vi "TCP Connection Manager.vi"(0 "TCP Ref":T1, 5 "Connection In":T3, 7 "Index":i32, 9 "Method":T5, 11 "error in (no error)":errorcluster, 12 "Properties In":T2) -> (3 "All Properties":T2[](array[typedef]), 4 "TCP Ref out":T1, 6 "Connection Out":T3, 8 "All Connections":T3[](array[typedef]), 10 "Number of Connections":i32, 14 "Properties out":T2, 15 "error out":errorcluster)   [LabVIEW 2013, in "J1939 Addon Shared.lvlib"]
doc: "This VI maintains the list of host connections."
uses:
  J1939 Addon Shared.lvlib
  stm_TCPConnectionMethod.ctl
  TCP/stm_TCP Connection Info.ctl
  _SubVIs/stm_MetaDataElement.ctl
  stm_TCPConnectionProperties.ctl
  J1939 Multi Packet Frame/Types/RQST Comm Lookup Table_Ref.ctl
  stm_ManagerStateVariables.ctl
  Engine/J1939 Addon Engine.lvlib
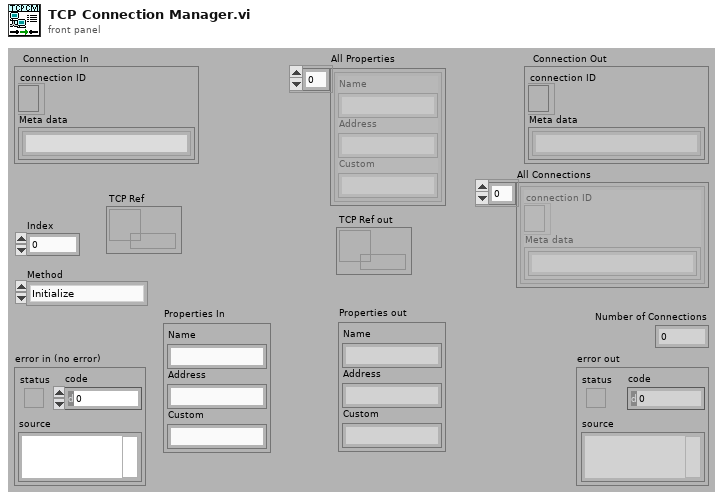
[diagram p1: front panel]
types:
  T1 = typedef "J1939 Addon Engine.lvlib/RQST Comm Lookup Table_Ref.ctl" = refnum<data-value>
  T2 = typedef "J1939 Addon Shared.lvlib/stm_TCPConnectionProperties.ctl" = cluster{"Name":string, "Address":string, "Custom":string}
  T3 = typedef "J1939 Addon Shared.lvlib/stm_TCP Connection Info.ctl" = cluster{"connection ID":refnum<k5>, "Meta data":T4[]}
  T4 = typedef "J1939 Addon Shared.lvlib/stm_MetaDataElement.ctl" = string
  T5 = typedef "J1939 Addon Shared.lvlib/stm_TCPConnectionMethod.ctl" = enum16{"Initialize", "Add Connection", "Set Properties", "Get Connection(s)", "Remove Connection", "Remove All Connections", "Get Connection Count"}
  T6 = typedef "J1939 Addon Shared.lvlib/stm_ManagerStateVariables.ctl" = cluster{"All Connections":T3[], "All Properties":T2[]}
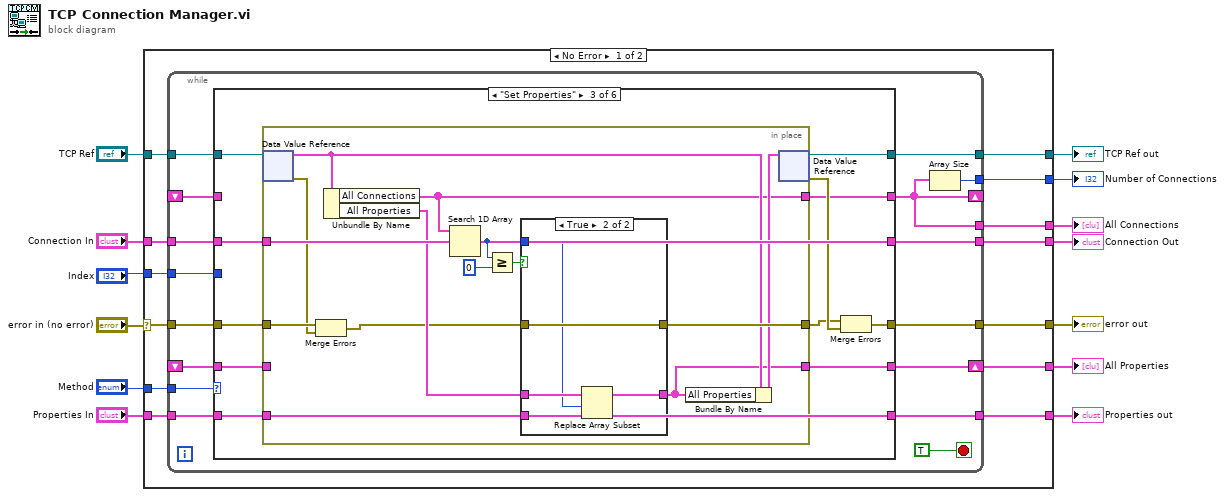
[diagram p0: block diagram]
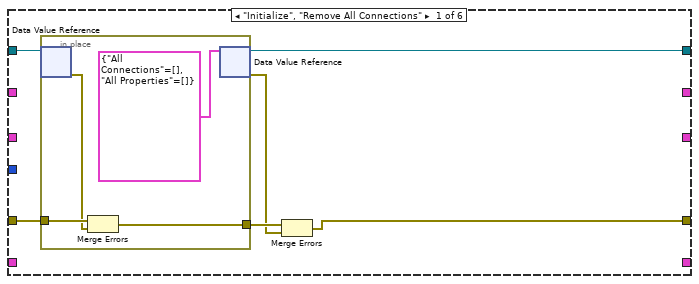
[diagram p2: hidden frame]
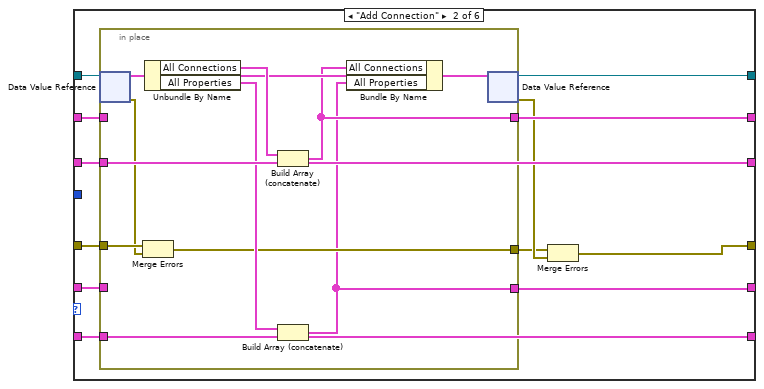
[diagram p3: hidden frame]
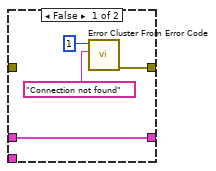
[diagram p4: hidden frame]
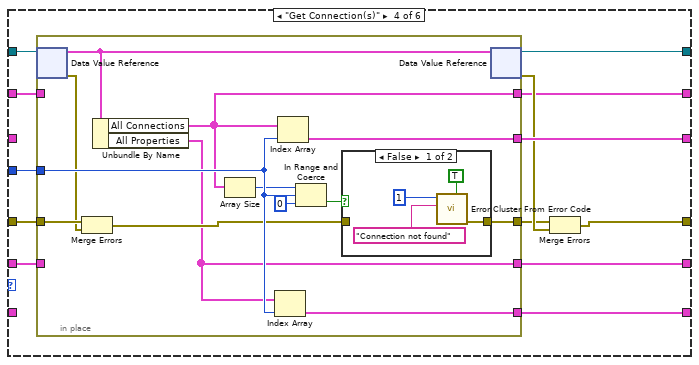
[diagram p5: hidden frame]
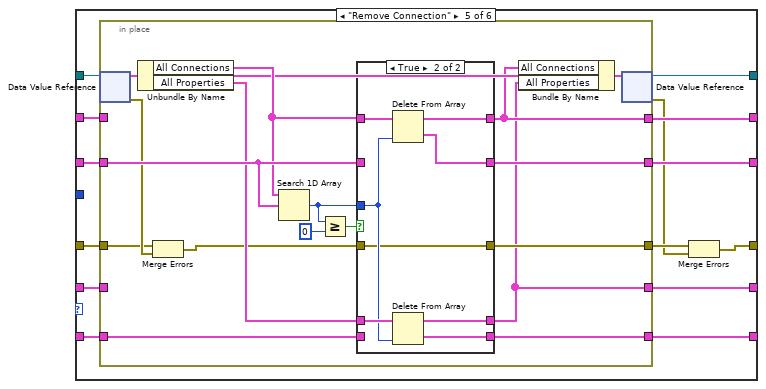
[diagram p7: hidden frame]
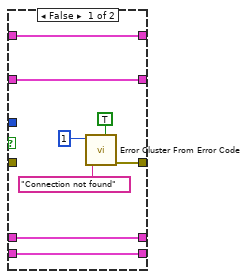
[diagram p8: hidden frame]
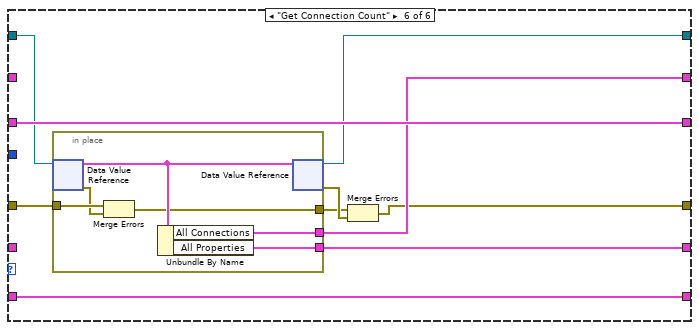
[diagram p9: hidden frame]
diagram:
  n1 = case shown="No Error" "error in (no error)" {
    selector: "error in (no error)" -> [w26 w206]
    tunnel: [w25 w206] -> w12
    tunnel: "Index" -> [w24 _]
    tunnel: "Method" -> [w23 _]
    tunnel: "Connection In" -> [w22 w205]
    tunnel: [w21 _] -> w8
    tunnel: [w20 _] -> w7
    tunnel: [w19 w205] -> w6
    tunnel: "Properties In" -> [w18 _]
    tunnel: [w17 _] -> w4
    tunnel: [w16 _] -> w3
    tunnel: "TCP Ref" -> [w15 w204]
    tunnel: [w14 w204] -> w1
    frame No Error {
      n2 = while {
        shift-right: [w34] -> _
        shift-left: _ -> [w41]
        tunnel: w26 -> [w40]
        tunnel: [w39] -> w25
        tunnel: w24 -> [w38]
        tunnel: w23 -> [w37]
        tunnel: w22 -> [w36]
        tunnel: [w35] -> w21
        tunnel: [w34] -> w20
        tunnel: [w33] -> w19
        shift-right: [w30] -> w17
        shift-left: _ -> [w32]
        tunnel: w18 -> [w31]
        tunnel: [w29] -> w16
        tunnel: w15 -> [w28]
        tunnel: [w27] -> w14
        stop <- TRUE stop-if-true
        n3 = case shown="\"Set Properties\"" w37 {
          tunnel: w41 -> [_ w64 _ w118 w154 _]
          tunnel: w36 -> [_ w62 w86 _ w150 w197]
          tunnel: [_ w63 w76 w111 w153 w194] -> w34
          tunnel: [_ w62 w86 w122 w152 w197] -> w33
          tunnel: [w44 w54 w80 w113 w143 w189] -> w39
          tunnel: w40 -> [w47 w57 w85 w117 w151 w192]
          tunnel: w38 -> [_ _ _ w119 _ _]
          tunnel: w32 -> [_ w61 w84 w121 w149 _]
          tunnel: w31 -> [_ w60 w83 _ w146 w196]
          tunnel: [_ w53 w77 w110 w148 w193] -> w30
          tunnel: [_ w60 w83 w120 w147 w196] -> w29
          tunnel: w28 -> [w48 w59 w82 w116 w145 w195]
          tunnel: [w43 w58 w78 w115 w144 w188] -> w27
          frame "Initialize", "Remove All Connections" {
            n4 = in-place {
              in-place-border: w47 -> [w51]
              in-place-border: [w49] -> w46
              n5 = in-place-dvr #1(w48) -> (w50:errorcluster)  [unwired: 1 out]
              n6 = Merge Errors(w51, w50) -> (w49:errorcluster)
              n7 = in-place-dvr #1(T6 {"All Connections"=[], "All Properties"=[]} ("data value")) -> (w43:T1, w45:errorcluster)
            }
            n8 = Merge Errors(w46, w45) -> (w44:errorcluster)
          }
          frame "Add Connection" {
            n9 = in-place {
              in-place-border: w64 -> [_]
              in-place-border: [w70] -> w63
              in-place-border: w62 -> [w75]
              in-place-border: w61 -> [_]
              in-place-border: w60 -> [w74]
              in-place-border: w57 -> [w68]
              in-place-border: [w66] -> w55
              in-place-border: [w65] -> w53
              n10 = in-place-dvr #2(w59) -> (w71:T6, w67:errorcluster)
              n11 = Merge Errors(w68, w67) -> (w66:errorcluster)
              n12 = Unbundle By Name(w71) -> ("All Connections"=w73:T3[], "All Properties"=w72:T2[])
              n13 = Build Array (concatenate)(w73, w75) -> (w70:T3[])
              n14 = Build Array (concatenate)(w72, w74) -> (w65:T2[])
              n15 = Bundle By Name(cluster=w71, "All Connections"=w70, "All Properties"=w65) -> (w69:T6)
              n16 = in-place-dvr #2(w69) -> (w58:T1, w56:errorcluster)
            }
            n17 = Merge Errors(w55, w56) -> (w54:errorcluster)
          }
          frame "Set Properties" {
            n18 = in-place {
              in-place-border: w86 -> [w99]
              in-place-border: w85 -> [w97]
              in-place-border: [w96] -> w79
              in-place-border: w84 -> [_]
              in-place-border: w83 -> [w94]
              in-place-border: [w88] -> w77
              in-place-border: [w87] -> w76
              n19 = in-place-dvr #3(w82) -> (w92:T6, w89:errorcluster)
              n20 = Merge Errors(w97, w89) -> (w90:errorcluster)
              n21 = Unbundle By Name(w92) -> ("All Connections"=w87:T3[], "All Properties"=w93:T2[])
              n22 = Search 1D Array(1D array=w87, element=w99) -> (index of element=w95:i32)  [unwired: 1 out]
              n23 = Greater Or Equal?(x=w95, y=0) -> (x >= y?=w98:bool)
              n24 = case shown="True" w98 {
                tunnel: w90 -> [_ w109]
                tunnel: [w101 w109] -> w96
                tunnel: w93 -> [w104 w108]
                tunnel: w95 -> [_ w107]
                tunnel: w94 -> [_ w106]
                tunnel: [w104 w105] -> w88
                frame False {
                  n25 = call <vilib>:"Error Cluster From Error Code.vi"("error message (\"\")"="Connection not found" ("source"), "error code (0)"=1 ("code")) -> ("error out"=w101:errorcluster)  [unwired: 2 in, 5 out]
                }
                frame True {
                  n26 = Replace Array Subset(array=w108, new element=w106, index=w107) -> (w105:T2[])
                }
              }
              n27 = Bundle By Name(cluster=w92, "All Properties"=w88) -> (w91:T6)
              n28 = in-place-dvr #3(w91) -> (w78:T1, w81:errorcluster)
            }
            n29 = Merge Errors(w79, w81) -> (w80:errorcluster)
          }
          frame "Get Connection(s)" {
            n30 = in-place {
              in-place-border: [w135] -> w122
              in-place-border: w121 -> [_]
              in-place-border: [w134] -> w120
              in-place-border: w119 -> [w133]
              in-place-border: w118 -> [_]
              in-place-border: w117 -> [w131]
              in-place-border: [w128] -> w112
              in-place-border: [w124] -> w111
              in-place-border: [w123] -> w110
              n31 = in-place-dvr #4(w116) -> (w127:T6, w125:errorcluster)
              n32 = Merge Errors(w131, w125) -> (w126:errorcluster)
              n33 = Unbundle By Name(w127) -> ("All Connections"=w124:T3[], "All Properties"=w123:T2[])
              n34 = Array Size(array=w124) -> (size(s)=w132:i32)
              n35 = Index Array(array=w123, index=w133) -> (element=w134:T2)
              n36 = Index Array(array=w124, index=w133) -> (element=w135:T3)
              n37 = In Range and Coerce(upper limit=w132, x=w133, lower limit=0) -> (In Range?=w130:bool)  [unwired: 1 out]
              n38 = case shown="False" w130 {
                tunnel: w126 -> [_ w140]
                tunnel: [w137 w140] -> w128
                frame False {
                  n39 = call <vilib>:"Error Cluster From Error Code.vi"("is warning? (False)"=TRUE, "error message (\"\")"="Connection not found" ("source"), "error code (0)"=1 ("code")) -> ("error out"=w137:errorcluster)  [unwired: 2 in, 4 out]
                }
                frame True {
                }
              }
              n40 = in-place-dvr #4(w127) -> (w115:T1, w114:errorcluster)
            }
            n41 = Merge Errors(w112, w114) -> (w113:errorcluster)
          }
          frame "Remove Connection" {
            n42 = in-place {
              in-place-border: w154 -> [_]
              in-place-border: [w159] -> w153
              in-place-border: [w168] -> w152
              in-place-border: [w167] -> w142
              in-place-border: w151 -> [w156]
              in-place-border: w150 -> [w166]
              in-place-border: w149 -> [_]
              in-place-border: [w158] -> w148
              in-place-border: [w165] -> w147
              in-place-border: w146 -> [w164]
              n43 = in-place-dvr #5(w145) -> (w161:T6, w157:errorcluster)
              n44 = Unbundle By Name(w161) -> ("All Connections"=w163:T3[], "All Properties"=w162:T2[])
              n45 = Merge Errors(w156, w157) -> (w155:errorcluster)
              n46 = Search 1D Array(1D array=w163, element=w166) -> (index of element=w171:i32)  [unwired: 1 out]
              n47 = Greater Or Equal?(x=w171, y=0) -> (x >= y?=w169:bool)
              n48 = case shown="True" w169 {
                tunnel: w163 -> [w179 w186]
                tunnel: w171 -> [_ w183]
                tunnel: [w179 w187] -> w159
                tunnel: [w178 w181] -> w168
                tunnel: [w175 w180] -> w167
                tunnel: w155 -> [_ w180]
                tunnel: w166 -> [w178 _]
                tunnel: w162 -> [w177 w185]
                tunnel: [w177 w184] -> w158
                tunnel: [w176 w182] -> w165
                tunnel: w164 -> [w176 _]
                frame False {
                  n49 = call <vilib>:"Error Cluster From Error Code.vi"("is warning? (False)"=TRUE, "error message (\"\")"="Connection not found" ("source"), "error code (0)"=1 ("code")) -> ("error out"=w175:errorcluster)  [unwired: 2 in, 4 out]
                }
                frame True {
                  n50 = Delete From Array(array=w186, index=w183) -> (deleted portion=w181:T3, array with subset deleted=w187:T3[])  [unwired: 1 in]
                  n51 = Delete From Array(array=w185, index=w183) -> (deleted portion=w182:T2, array with subset deleted=w184:T2[])  [unwired: 1 in]
                }
              }
              n52 = Bundle By Name(cluster=w161, "All Connections"=w159, "All Properties"=w158) -> (w160:T6)
              n53 = in-place-dvr #5(w160) -> (w144:T1, w141:errorcluster)
            }
            n54 = Merge Errors(w142, w141) -> (w143:errorcluster)
          }
          frame "Get Connection Count" {
            n55 = in-place {
              in-place-border: [w203] -> w194
              in-place-border: [w202] -> w193
              in-place-border: w192 -> [w200]
              in-place-border: [w198] -> w190
              n56 = in-place-dvr #6(w195) -> (w201:T6, w199:errorcluster)
              n57 = Merge Errors(w200, w199) -> (w198:errorcluster)
              n58 = Unbundle By Name(w201) -> ("All Connections"=w203:T3[], "All Properties"=w202:T2[])
              n59 = in-place-dvr #6(w201) -> (w188:T1, w191:errorcluster)
            }
            n60 = Merge Errors(w190, w191) -> (w189:errorcluster)
          }
        }
        n61 = Array Size(array=w34) -> (size(s)=w35:i32)
      }
    }
    frame Error {
    }
  }
  "error out" <- w12
  "Number of Connections" <- w8
  "All Connections" <- w7
  "Connection Out" <- w6
  "All Properties" <- w4
  "Properties out" <- w3
  "TCP Ref out" <- w1
